vi "poly_signalling_write_multi_2.vi"(6 "modes (Sgnl)":T1(array[ring]), 8 "error in (no error)":errorcluster, 9 "values":variant[](array[variant]), 10 "control names":string[](array[string]), 11 "vi reference":refnum<vi>) -> (0 "error out":errorcluster, 2 "control refs":refnum<vi>[](array[refnum]), 3 "vi reference out":refnum<vi>, 4 "found?":bool[](array[boolean]))   [LabVIEW 2015, in "_ref_tools_polys.lvlib"]
uses:
  _ref_tools_polys.lvlib
  poly_control_ref_from_name_multi.vi
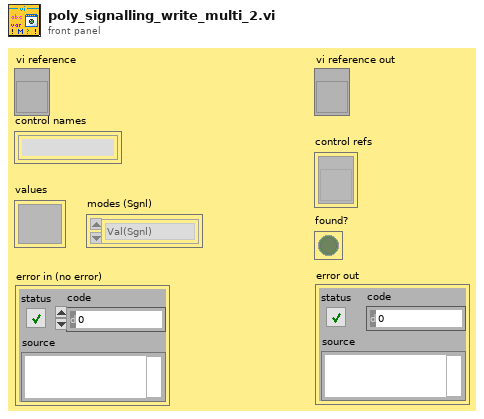
[diagram p1: front panel]
types:
  T1 = enum16{"Val", "Val(Sgnl)", "Val(Undo)", "Method"}[]
  T2 = enum16{"Val", "Val(Sgnl)", "Val(Undo)", "Method"}
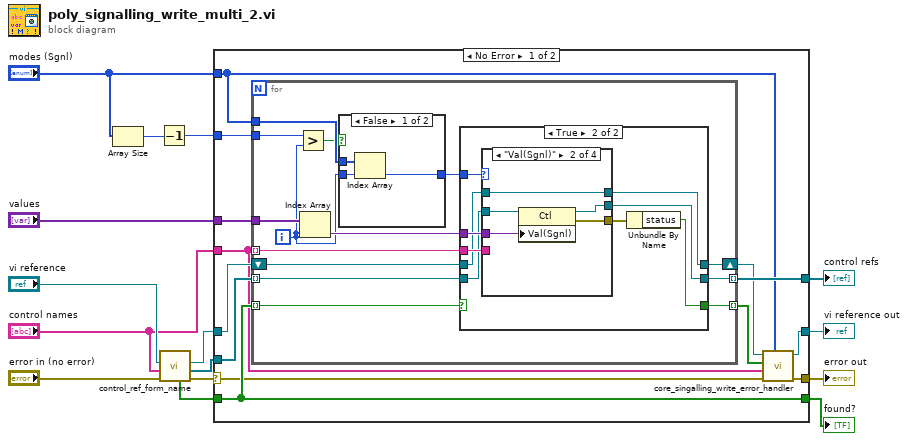
[diagram p0: block diagram]
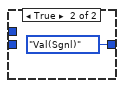
[diagram p2: hidden frame]
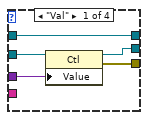
[diagram p4: hidden frame]
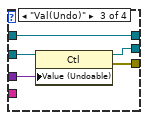
[diagram p5: hidden frame]
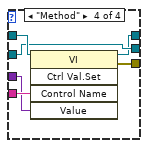
[diagram p6: hidden frame]
diagram:
  n1 = Array Size(array="modes (Sgnl)") -> (size(s)=w4:i32)
  n2 = Decrement(x=w4) -> (x-1=w3:i32)
  n3 = call-poly "control_ref_form_name.vi"("error in (no error)"="error in (no error)", "control names"="control names", "vi ref"="vi reference") -> ("error out"=w2:errorcluster, "ctrl refs"=w11:refnum<vi>[], "vi ref dup"=w10:refnum<vi>, "found?"=w6:bool[])  [unwired: 5 in]
  n4 = case shown="No Error" w2 {
    selector: w2 -> [w22 w83]
    tunnel: [w21 w83] -> w15
    tunnel: [w17 w81] -> w14
    tunnel: w11 -> [w28 w82]
    tunnel: w10 -> [w27 w81]
    tunnel: "control names" -> [w19 _]
    tunnel: "values" -> [w26 _]
    tunnel: [w25 w82] -> w7
    tunnel: w6 -> [w23 w80]
    tunnel: "modes (Sgnl)" -> [w16 _]
    tunnel: w3 -> [w24 _]
    tunnel: [w23 w80] -> w1
    frame No Error {
      n5 = for {
        tunnel: w16 -> [w34]
        tunnel: [w42] -> w25 mode=indexing
        tunnel: w28 -> [w36] mode=indexing
        tunnel: w19 -> [w39] mode=indexing
        shift-right: [w41] -> w18
        shift-left: w27 -> [w40]
        tunnel: w26 -> [w38]
        tunnel: w23 -> [w35] mode=indexing
        tunnel: w24 -> [w31]
        tunnel: [w29] -> w20 mode=indexing
        i -> [w32]
        n6 = Greater?(x=w31, y=w32) -> (0:w30:bool)
        n7 = Index Array(array=w38, index=w32) -> (element=w37:variant)
        n8 = case shown="False" w30 {
          tunnel: w34 -> [w45 _]
          tunnel: w32 -> [w44 _]
          tunnel: [w43 T2."Val(Sgnl)" ("mode (Sgnl)")] -> w33
          frame False {
            n9 = Index Array(array=w45, index=w44) -> (element=w43:T2)
          }
          frame True {
          }
        }
        n10 = case shown="True" w35 {
          selector: w35 -> [w47 _]
          tunnel: w37 -> [_ w58]
          tunnel: w33 -> [_ w57]
          tunnel: [w48 w56] -> w42
          tunnel: [w49 w55] -> w41
          tunnel: w39 -> [_ w54]
          tunnel: w40 -> [w49 w53]
          tunnel: w36 -> [w48 w52]
          tunnel: [w47 w50] -> w29
          frame False {
          }
          frame True {
            n11 = case shown="\"Val(Sgnl)\"" w57 {
              tunnel: w52 -> [w63 w65 w72 w77]
              tunnel: w58 -> [w62 w68 w73 w74]
              tunnel: [w61 w67 w69 w78] -> w51
              tunnel: [w60 w66 w71 w77] -> w56
              tunnel: w53 -> [w59 w64 w70 w79]
              tunnel: [w59 w64 w70 w76] -> w55
              tunnel: w54 -> [_ _ _ w75]
              frame "Val" {
                n12 = property class="Ctl"(reference=w63, "Value"=w62) -> (reference out=w60:refnum<vi>, error out=w61:errorcluster)  [unwired: 1 in]
              }
              frame "Val(Sgnl)" {
                n13 = property class="Ctl"(reference=w65, "Val(Sgnl)"=w68) -> (reference out=w66:refnum<vi>, error out=w67:errorcluster)  [unwired: 1 in]
              }
              frame "Val(Undo)" {
                n14 = property class="Ctl"(reference=w72, "Value (Undoable)"=w73) -> (reference out=w71:refnum<vi>, error out=w69:errorcluster)  [unwired: 1 in]
              }
              frame "Method" {
                n15 = invoke class="VI" method="Ctrl Val.Set"(reference=w79, "Control Name"=w75, "Value"=w74) -> (reference out=w76:refnum<vi>, error out=w78:errorcluster)  [unwired: 2 in, 3 out]
              }
            }
            n16 = Unbundle By Name(w51) -> ("status"=w50:bool)
          }
        }
      }
      n17 = call "core_singalling_write_error_handler.vi"("modes (Sgnl)"=w16, "error in"=w22, "control names"=w19, "error?"=w20, "vi ref"=w18) -> ("error out"=w21:errorcluster, "vi ref dup"=w17:refnum<vi>)  [unwired: 5 in]
    }
    frame Error {
    }
  }
  "error out" <- w15
  "vi reference out" <- w14
  "found?" <- w1
  "control refs" <- w7
